vi "亚为噪音报告设置与初始化.vi"() -> (3 "appended path":path caption="path")   [LabVIEW 2011]
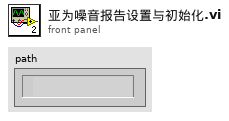
[diagram p1: front panel]
types:
  T1 = cluster{"测试人员":string, "项目名称":string, "部门":string, "测试对象":string, "测试条件":string, "数量":string, "温度":string, "湿度":string, "环境噪音":string}
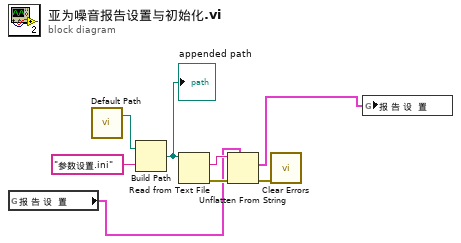
[diagram p0: block diagram]
diagram:
  n1 = global read "全局变量.vi" "报 告 设  置"() -> (w2:T1)
  n2 = call "Default Path.vi"() -> ("Default Path data"=w5:path)  [unwired: 3 in, 1 out]
  n3 = Build Path(base path=w5, name or relative path="参数设置.ini" ("名称或相对路径")) -> (appended path=w3:path)
  "appended path" <- w3
  n4 = Read from Text File(file (use dialog)=w3) -> (text=w7:string, error out=w8:errorcluster)  [unwired: 3 in, 2 out]
  n5 = Unflatten From String(type=w2, binary string=w7, error in (no error)=w8) -> (value=w1:T1, error out=w4:errorcluster)  [unwired: 2 in, 1 out]
  n6 = call <vilib>:"Clear Errors.vi"("error in (no error)"=w4) -> ()  [unwired: 5 in, 2 out]
  n7 = global write "全局变量.vi" "报 告 设  置"(w1) -> ()
